vi "Sleep HL -- subVI.vi"(8 "error in (no error)":errorcluster, 10 "User events":T1, 11 "event data":bool) -> (0 "error out":errorcluster)   [LabVIEW 2020, in "NI DAQ.lvlib"]
uses:
  NI DAQ.lvlib
  Task list.ctl
  Continuous aquisition params.ctl
  Controls/Acuisition type --typedef.ctl
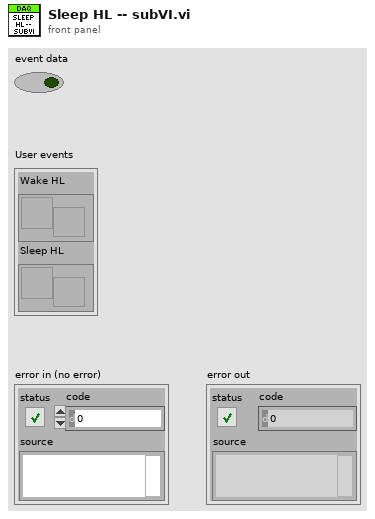
[diagram p1: front panel]
types:
  T1 = cluster{"Wake HL":refnum<user-event>, "Sleep HL":refnum<user-event>}
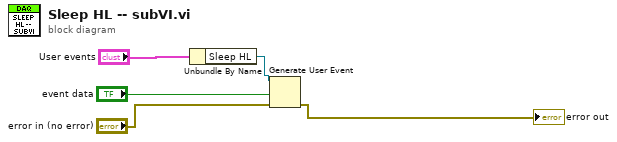
[diagram p0: block diagram]
diagram:
  n1 = Unbundle By Name("User events") -> ("Sleep HL"=w4:refnum<user-event>)
  n2 = Generate User Event(user event=w4, event data cluster="event data", error in="error in (no error)") -> (error out=→"error out":errorcluster)  [unwired: 1 in, 1 out]
